vi "getAxisStatus.vi"(8 "error in":errorcluster, 10 "axis":i32, 11 "connection ID":refnum<k5>) -> (0 "error out":errorcluster, 1 "status":T1, 2 "axis":i32, 3 "connection ID":refnum<k5>)   [LabVIEW 2016]
panel:
  in  "cluster":T1
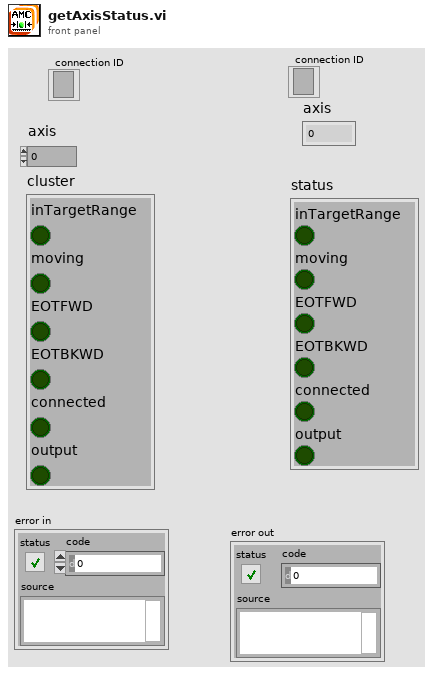
[diagram p1: front panel]
types:
  T1 = cluster{"inTargetRange":bool, "moving":bool, "EOTFWD":bool, "EOTBKWD":bool, "connected":bool, "output":bool}
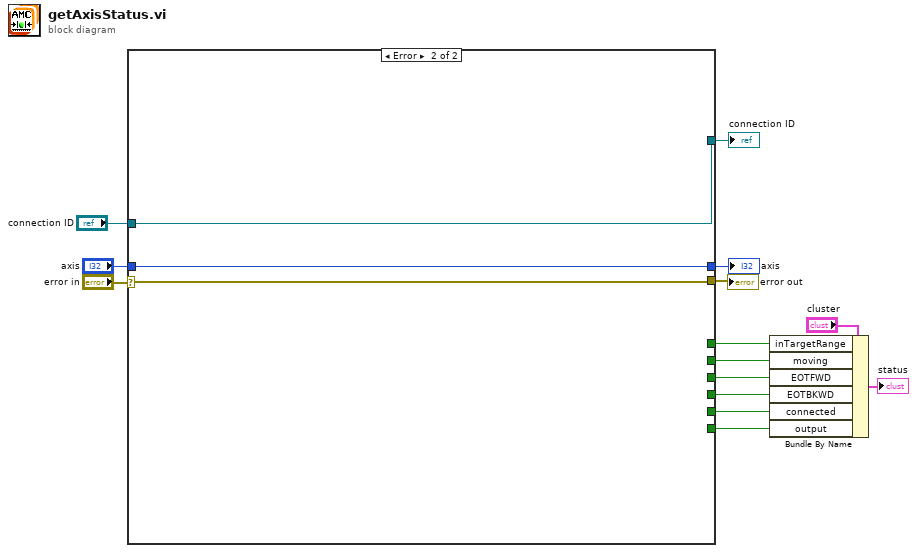
[diagram p0: block diagram]
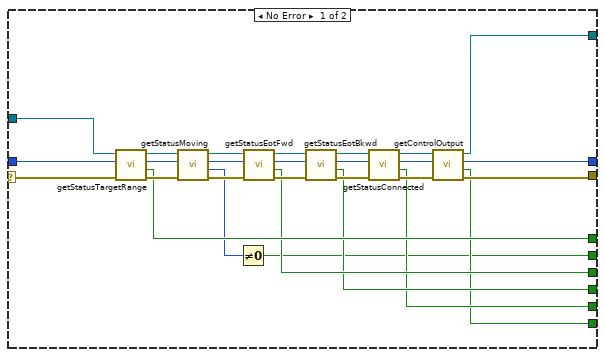
[diagram p2: hidden frame]
diagram:
  n1 = case shown="Error" "error in" {
    selector: "error in" -> [w42 w45]
    tunnel: [w36 w45] -> w14
    tunnel: [w29 w44] -> w13
    tunnel: "connection ID" -> [w35 w44]
    tunnel: "axis" -> [w28 w43]
    tunnel: [w22 _] -> w8
    tunnel: [w21 _] -> w7
    tunnel: [w20 _] -> w6
    tunnel: [w19 _] -> w5
    tunnel: [w18 _] -> w4
    tunnel: [w17 w43] -> w2
    tunnel: [w15 _] -> w1
    frame No Error {
      n2 = call "getStatusTargetRange.vi"("error in"=w42, "axis"=w28, "connection ID"=w35) -> ("error out"=w41:errorcluster, "boolean"=w22:bool, "axis_out"=w27:i32, "connection ID"=w34:refnum<k5>)  [unwired: 5 in]
      n3 = call "getStatusMoving.vi"("error in"=w41, "axis"=w27, "connection ID"=w34) -> ("error out"=w40:errorcluster, "status"=w16:i32, "axis_out"=w26:i32, "connection ID"=w33:refnum<k5>)  [unwired: 5 in]
      n4 = Not Equal To 0?(x=w16) -> (x != 0?=w15:bool)
      n5 = call "getStatusEotFwd.vi"("error in"=w40, "axis"=w26, "connection ID"=w33) -> ("error out"=w39:errorcluster, "boolean"=w21:bool, "axis_out"=w25:i32, "connection ID"=w32:refnum<k5>)  [unwired: 5 in]
      n6 = call "getStatusEotBkwd.vi"("error in"=w39, "axis"=w25, "connection ID"=w32) -> ("error out"=w38:errorcluster, "boolean"=w20:bool, "axis_out"=w24:i32, "connection ID"=w31:refnum<k5>)  [unwired: 5 in]
      n7 = call "getStatusConnected.vi"("error in"=w38, "axis"=w24, "connection ID"=w31) -> ("error out"=w37:errorcluster, "boolean"=w19:bool, "axis_out"=w23:i32, "connection ID"=w30:refnum<k5>)  [unwired: 5 in]
      n8 = call "getControlOutput.vi"("error in"=w37, "axis"=w23, "connection ID"=w30) -> ("error out"=w36:errorcluster, "boolean"=w18:bool, "axis_out"=w17:i32, "connection ID"=w29:refnum<k5>)  [unwired: 5 in]
    }
    frame Error {
    }
  }
  "error out" <- w14
  "connection ID" <- w13
  "axis" <- w2
  n9 = Bundle By Name(cluster="cluster", "inTargetRange"=w8, "moving"=w1, "EOTFWD"=w7, "EOTBKWD"=w6, "connected"=w5, "output"=w4) -> (→"status":T1)
